vi "Geometry.vi"() -> ()   [LabVIEW 2018]
uses:
  <vilib>/Analysis/coordinate.llb/Euler Rotation Order.ctl
  <vilib>/imath/engines/lvmath2/RunTimeEngine/NodeEndStatement/NIMS_NodeEndStatement_Output.vi
  <instcachedir>/0/NIMS_NodeEndStatement_Output_53EC0D466D134D7ABD903AC30B43404B.lvgen/NIMS_NodeEndStatement_Output_53EC0D466D134D7ABD903AC30B43404B_005.vi
  <instcachedir>/0/NIMS_NodeEndStatement_Output_53EC0D466D134D7ABD903AC30B43404B.lvgen/NIMS_NodeEndStatement_Output_53EC0D466D134D7ABD903AC30B43404B_002.vi
  <vilib>/imath/engines/lvmath2/RunTimeEngine/ErrorHandling/NIMS_Finalize Error.vi
  <vilib>/imath/engines/lvmath2/RunTimeEngine/IndexRead/NIMS V(S).vi
  <instcachedir>/0/NIMS V(S)_0488751826AF41519A22953C041130DC.lvgen/NIMS V(S)_0488751826AF41519A22953C041130DC_000.vi
  <vilib>/imath/engines/lvmath2/RunTimeEngine/ErrorHandling/NIMS_Create Error From Enums.vi
  <vilib>/imath/engines/lvmath2/RunTimeEngine/ArithmeticOperatorToken/NIMS_ArithmeticOperator_multmx(M,CV)-internal.vi
  <instcachedir>/0/NIMS_ArithmeticOperator_multmx(M,CV)-internal_5287250D8D1D4A3E9F77F5DF08D432E0.lvgen/NIMS_ArithmeticOperator_multmx(M,CV)-internal_5287250D8D1D4A3E9F77F5DF08D432E0_001.vi
  <vilib>/imathl/engines/lvmath/Functions/Error Handling/Create Error.vi
  <vilib>/imath/engines/lvmath2/RunTimeEngine/ArithmeticOperatorToken/NIMS_ArithmeticOperator_multmx.vi
  <instcachedir>/0/NIMS_ArithmeticOperator_multmx_622CA76F9646436AB036D42A9A1CE0E6.lvgen/NIMS_ArithmeticOperator_multmx_622CA76F9646436AB036D42A9A1CE0E6_004.vi
  <vilib>/imath/engines/lvmath2/RunTimeEngine/ArithmeticOperatorToken/NIMS_ArithmeticOperator_multmx(M,CV).vi
  <instcachedir>/0/NIMS_ArithmeticOperator_multmx(M,CV)_2F1CD6A2FE4F4213A4AD1C901C2750F5.lvgen/NIMS_ArithmeticOperator_multmx(M,CV)_2F1CD6A2FE4F4213A4AD1C901C2750F5_000.vi
  <vilib>/imath/engines/lvmath2/RunTimeEngine/ArithmeticOperatorToken/NIMS_ArithmeticOperator_minus.vi
  <instcachedir>/0/NIMS_ArithmeticOperator_minus_C4D0373119CC411691B2E50DF2E09F22.lvgen/NIMS_ArithmeticOperator_minus_C4D0373119CC411691B2E50DF2E09F22_002.vi
  <vilib>/imath/engines/lvmath2/RunTimeEngine/IndexRead/NIMS M(S,S).vi
  <instcachedir>/0/NIMS M(S,S)_AC51E74150A542F7991B9634C66F3096.lvgen/NIMS M(S,S)_AC51E74150A542F7991B9634C66F3096_000.vi
  <instcachedir>/0/NIMS_NodeEndStatement_Output_53EC0D466D134D7ABD903AC30B43404B.lvgen/NIMS_NodeEndStatement_Output_53EC0D466D134D7ABD903AC30B43404B_001.vi
  <vilib>/imath/engines/lvmath2/RunTimeEngine/ArithmeticOperatorToken/NIMS_ArithmeticOperator_plus.vi
  <instcachedir>/0/NIMS_ArithmeticOperator_plus_DE670E32103C4C10ADF2A97367172B30.lvgen/NIMS_ArithmeticOperator_plus_DE670E32103C4C10ADF2A97367172B30_003.vi
  <instcachedir>/0/NIMS_NodeEndStatement_Output_53EC0D466D134D7ABD903AC30B43404B.lvgen/NIMS_NodeEndStatement_Output_53EC0D466D134D7ABD903AC30B43404B_004.vi
  <vilib>/imath/engines/lvmath2/RunTimeEngine/BuiltInFunctions/cross/NIMS_cross(GV,GV).vi
  <instcachedir>/0/NIMS_cross(GV,GV)_8E551EB9DC304C30866B49598818C259.lvgen/NIMS_cross(GV,GV)_8E551EB9DC304C30866B49598818C259_000.vi
  <vilib>/imath/engines/lvmath2/RunTimeEngine/BuiltInFunctions/inv/NIMS_inv(GM).vi
  <instcachedir>/0/NIMS_inv(GM)_A6DF8FE880224208AACFE4CF9F659502.lvgen/NIMS_inv(GM)_A6DF8FE880224208AACFE4CF9F659502_000.vi
  <vilib>/imath/engines/lvmath2/RunTimeEngine/ErrorHandling/NIMS_Error From Error Code.vi
  <vilib>/imath/engines/lvmath2/RunTimeEngine/BuiltInFunctions/cross/NIMS_cross(GM,GM,I32).vi
  <instcachedir>/0/NIMS_cross(GM,GM,I32)_0F6D45CF7D834A0BB6695B819A7F63BC.lvgen/NIMS_cross(GM,GM,I32)_0F6D45CF7D834A0BB6695B819A7F63BC_000.vi
  <vilib>/imath/engines/lvmath2/RunTimeEngine/IndexRead/NIMS M(S).vi
  <instcachedir>/0/NIMS M(S)_B826C018497E4940AE96BD27B540B6FB.lvgen/NIMS M(S)_B826C018497E4940AE96BD27B540B6FB_000.vi
  <vilib>/imath/engines/lvmath2/RunTimeEngine/BuiltInFunctions/norm/NIMS_norm(GM,DBL).vi
  <instcachedir>/0/NIMS_norm(GM,DBL)_14A9435485184B5E92336AF75A728284.lvgen/NIMS_norm(GM,DBL)_14A9435485184B5E92336AF75A728284_000.vi
  <vilib>/imath/engines/lvmath2/RunTimeEngine/IndexReplace/NIMS M(S,S)=S.vi
  <instcachedir>/0/NIMS M(S,S)=S_5DAF17B45D8A4C8588C7CF468644990A.lvgen/NIMS M(S,S)=S_5DAF17B45D8A4C8588C7CF468644990A_000.vi
  <vilib>/imath/engines/lvmath2/RunTimeEngine/NodeEndStatement/NIMS_NodeEndStatement_Get Vector.vi
  <instcachedir>/0/NIMS_NodeEndStatement_Get Vector_329D0992E87F49F089135171B7FC9327.lvgen/NIMS_NodeEndStatement_Get Vector_329D0992E87F49F089135171B7FC9327_001.vi
  <vilib>/imath/engines/lvmath/Functions/Error Handling/MergeErrorsWrapper.vi
  <vilib>/Analysis/NI_AALPro.lvlib
panel:
  out "rmg":dbl[](array[numeric])
  out "er 3":dbl(graph)
  out "er2":dbl(graph)
  out "er1":dbl(graph)
  out "Waveform Chart 3":dbl(graph)
  out "Waveform Chart 2":dbl(graph)
  out "Waveform Chart":dbl(graph)
  in  "Simulation Time(sec)":dbl
  in  "Physical Parameters":T1
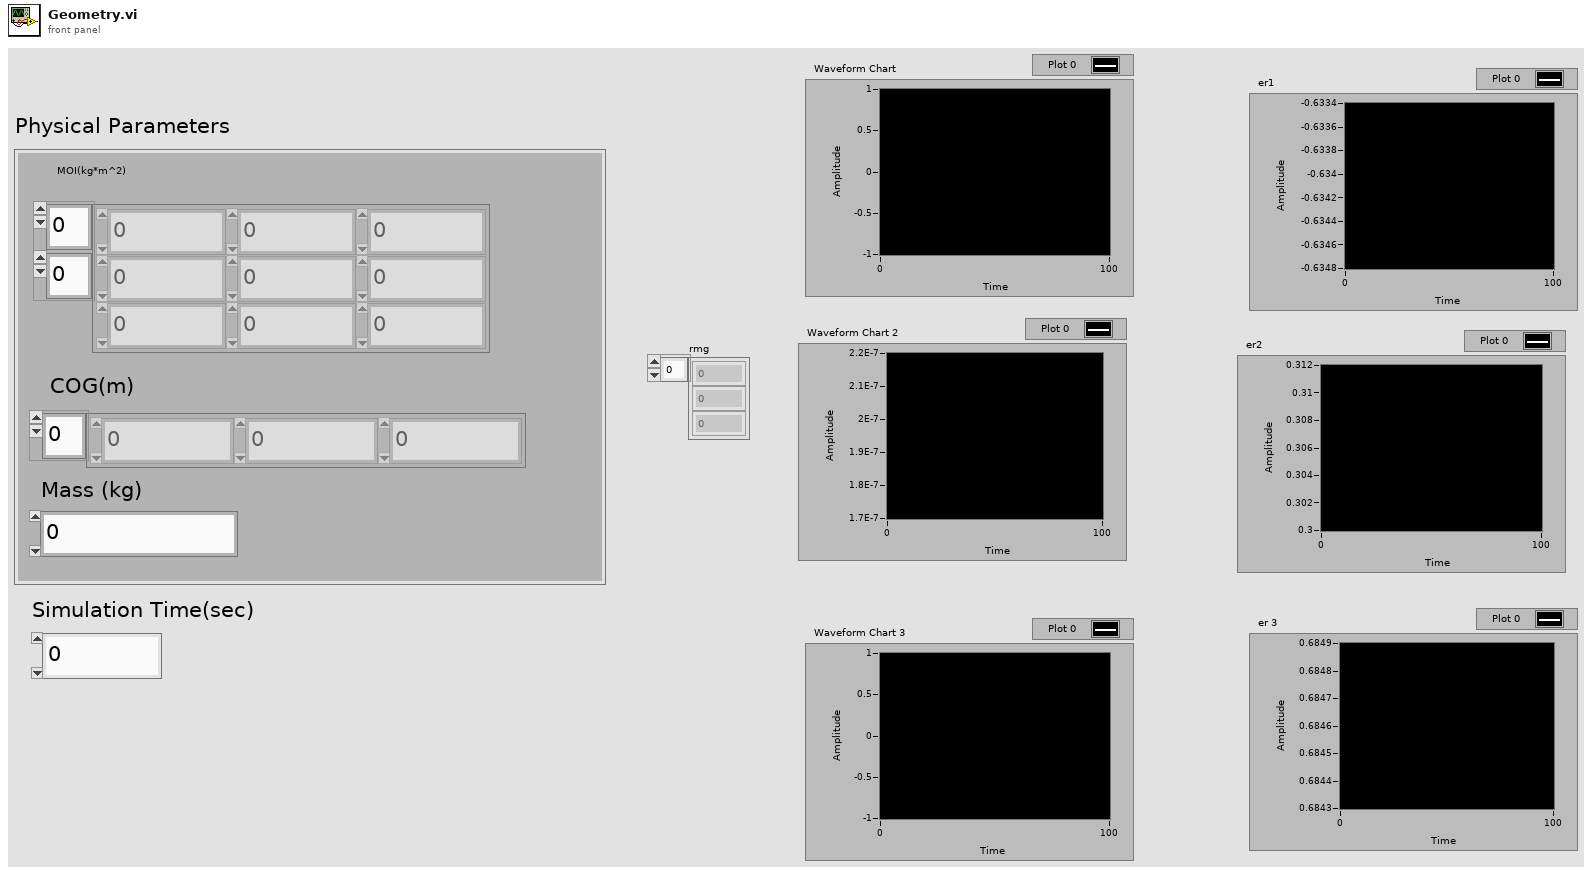
[diagram p1: front panel]
types:
  T1 = cluster{"Mass (kg)":dbl, "COG(m)":dbl[], "MOI(kg*m^2)":dbl[][]}
  T2 = typedef "NI_AALPro.lvlib/Euler Rotation Order.ctl" = u16
  T3 = cluster{"Direction Cosines":dbl[][], "Wd":dbl[], "W_dot_d":dbl[]}
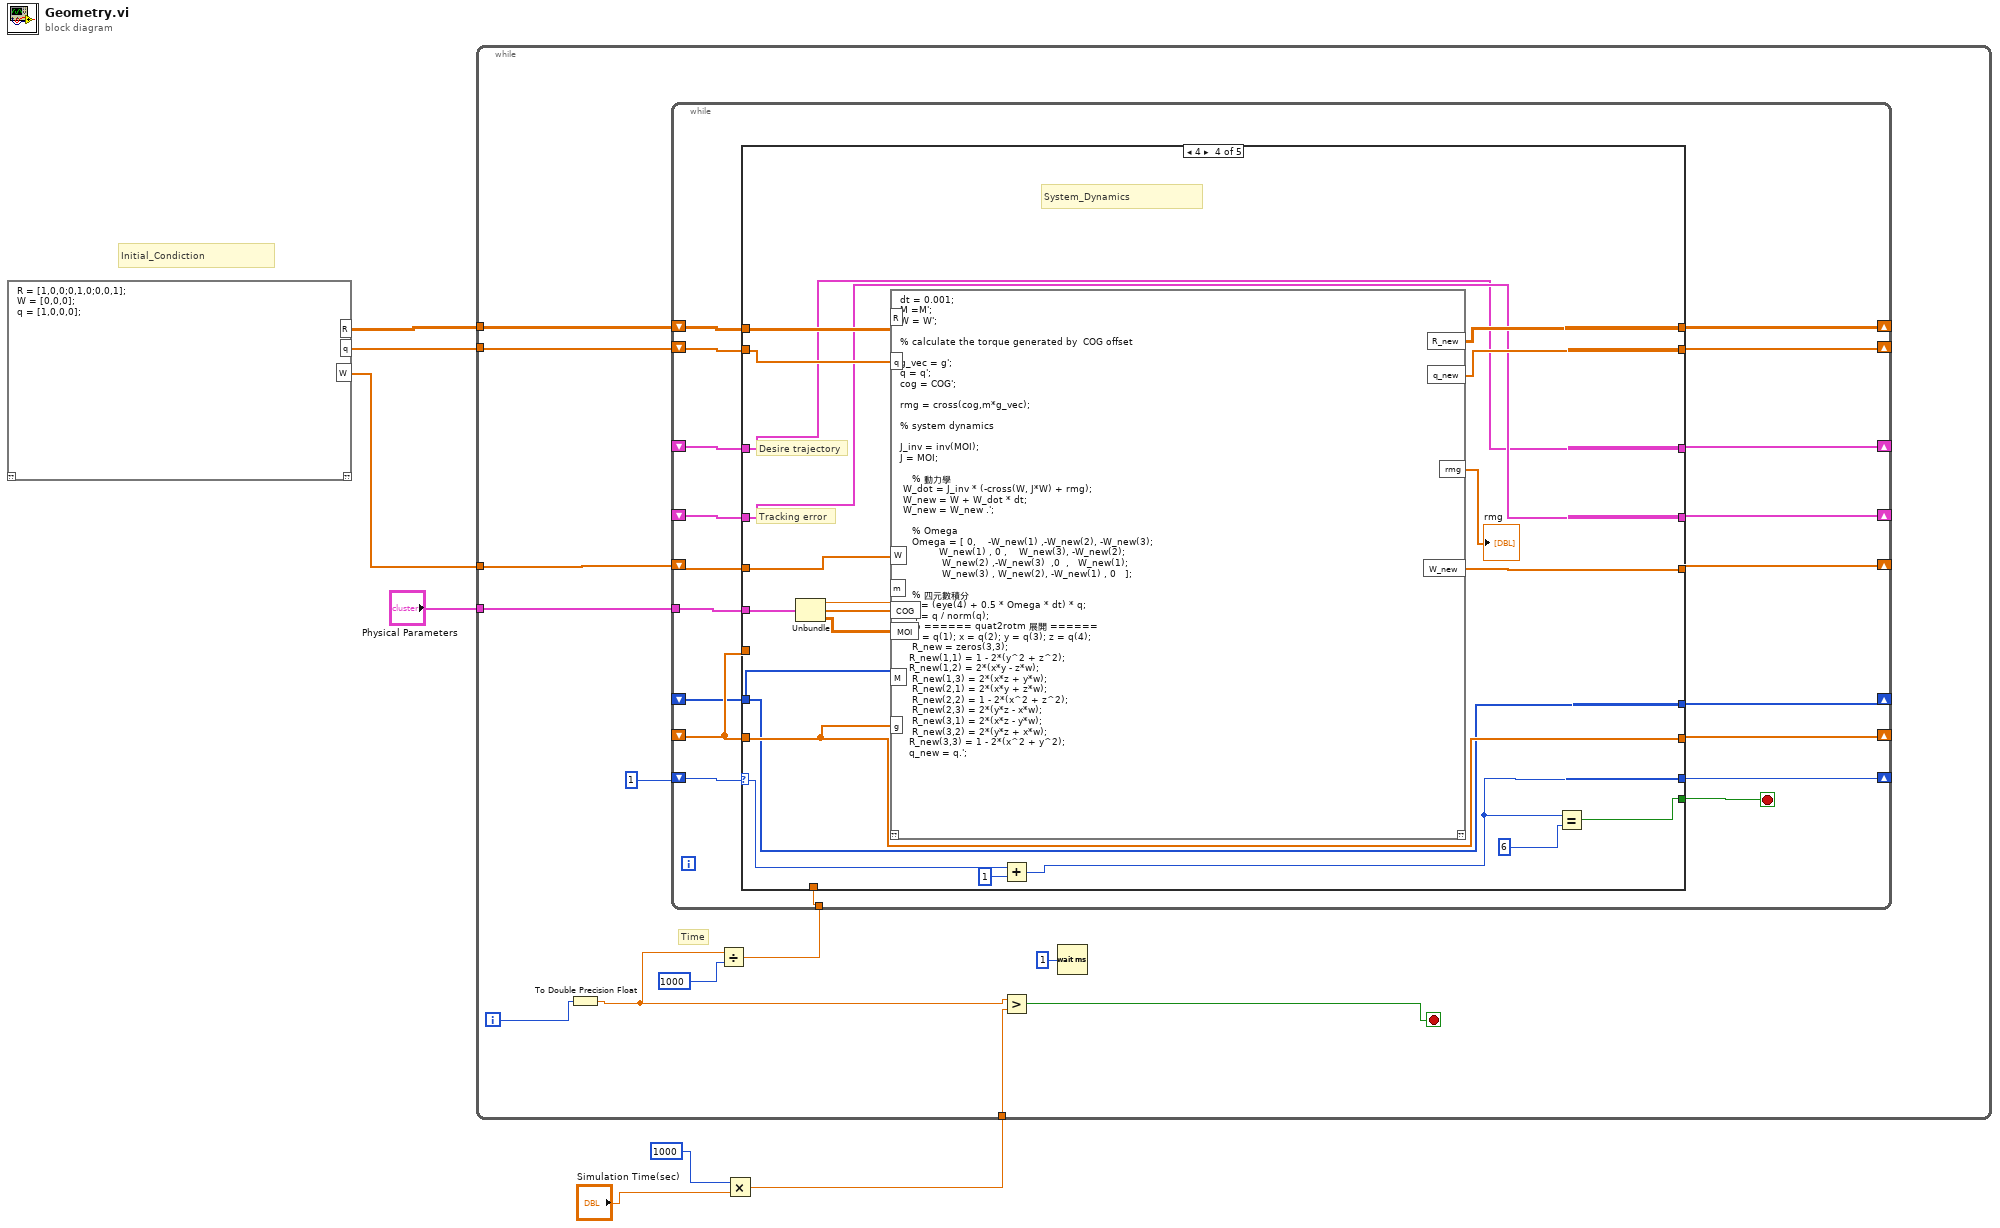
[diagram p0: block diagram]
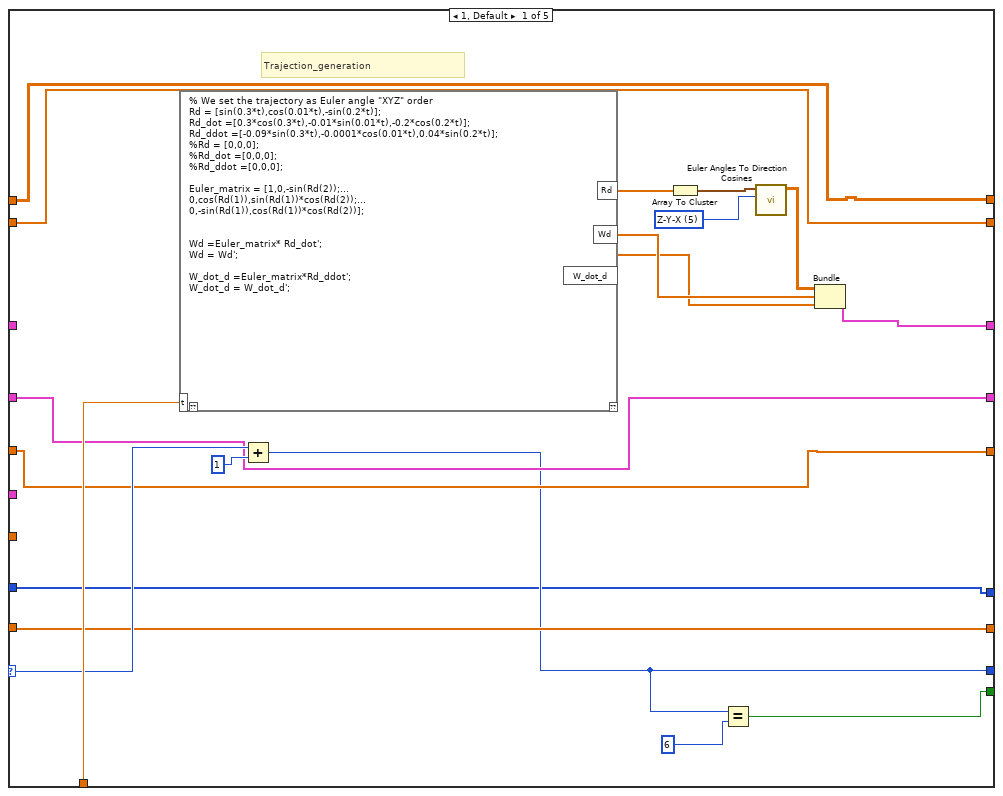
[diagram p2: hidden frame]
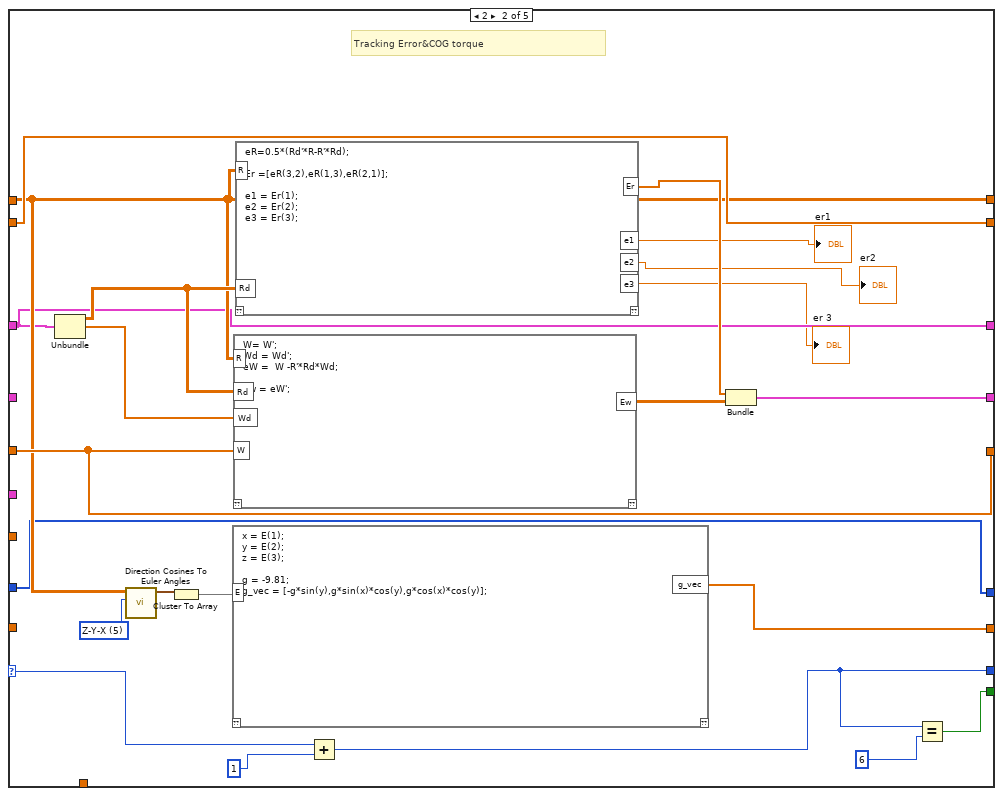
[diagram p3: hidden frame]
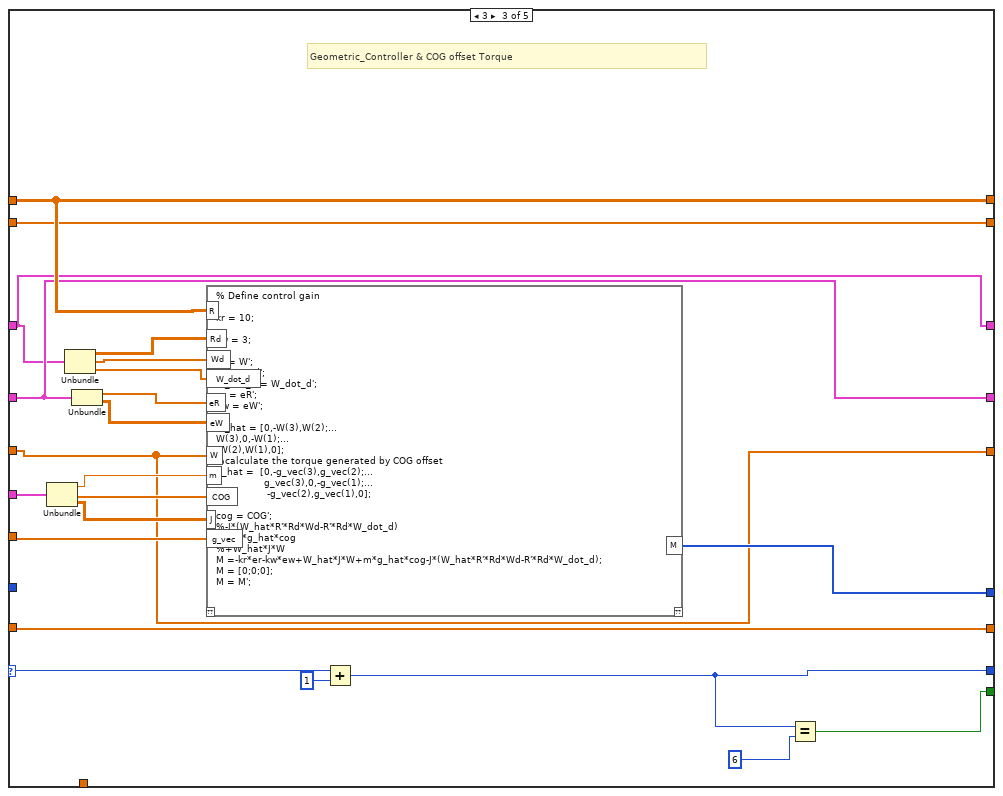
[diagram p4: hidden frame]
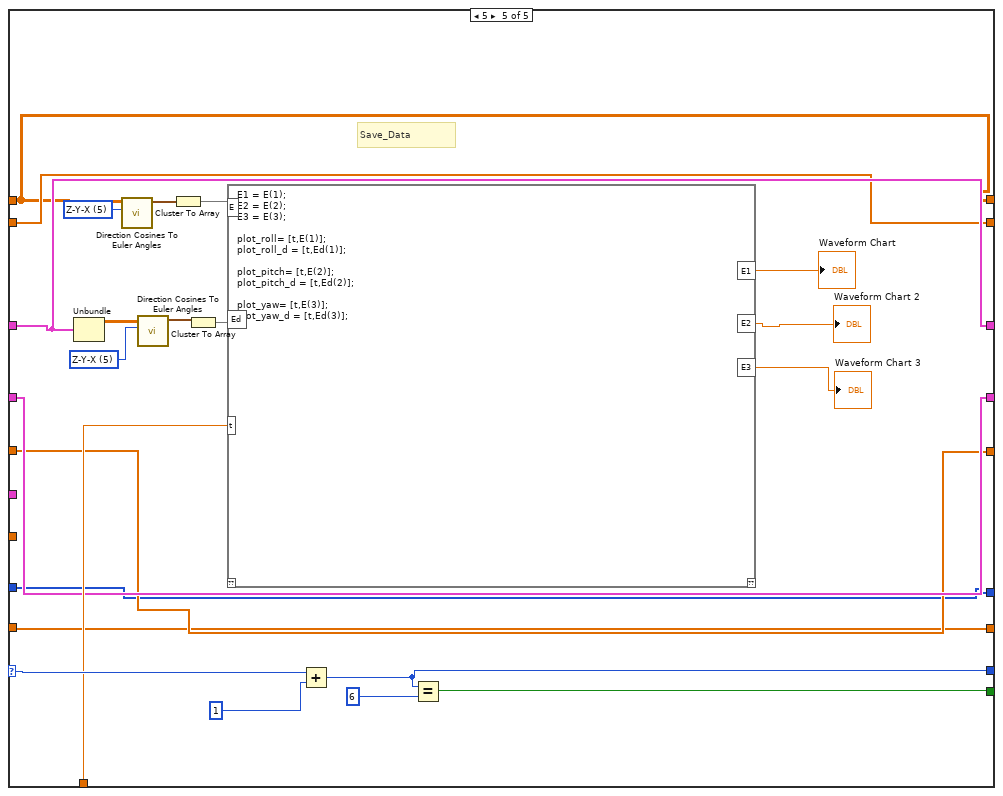
[diagram p5: hidden frame]
diagram:
  # "Initial_Condiction"
  n1 = mathscript code="R = [1,0,0;0,1,0;0,0,1];\nW = [0,0,0];\nq = [1,0,0,0];"() -> ("R"=w4:dbl[][], "W"=w3:dbl[], "q"=w1:dbl[])  [unwired: 1 in, 1 out]
  n2 = Multiply(x=1000, y="Simulation Time(sec)") -> (x*y=w5:dbl)
  n3 = while {
    tunnel: w5 -> [w17]
    tunnel: w4 -> [w12]
    tunnel: w3 -> [w11]
    tunnel: "Physical Parameters" -> [w10]
    tunnel: w1 -> [w9]
    i -> [w15]
    stop <- w18 stop-if-true
    # "Time"
    n4 = To Double Precision Float(number=w15) -> (double precision float=w13:dbl)
    n5 = Divide(x=w13, y=1000) -> (x/y=w14:dbl)
    n6 = while {
      shift-right: [w36] -> _
      shift-left: 1 -> [w38]
      tunnel: w14 -> [w37]
      shift-right: [w35] -> _
      shift-left: _ -> [w34]
      shift-right: [w33] -> _
      shift-left: _ -> [w32]
      shift-right: [w29] -> _
      shift-left: w12 -> [w31]
      shift-right: [w28] -> _
      shift-left: w11 -> [w30]
      shift-right: [w27] -> _
      shift-left: _ -> [w26]
      tunnel: w10 -> [w25]
      shift-right: [w24] -> _
      shift-left: _ -> [w23]
      shift-right: [w21] -> _
      shift-left: w9 -> [w22]
      stop <- w20 stop-if-true
      n7 = case shown="4" w38 {
        selector: w38 -> [w53 w262 w580 w896 w1606]
        tunnel: w37 -> [w57 _ _ _ w1595]
        tunnel: [w54 w255 w576 w889 w1594] -> w35
        tunnel: [w42 w253 w574 w886 w1587] -> w36
        tunnel: w34 -> [_ w255 w576 w889 w1594]
        tunnel: [w45 w264 w577 w890 w1593] -> w33
        tunnel: w32 -> [w45 _ w577 w890 w1593]
        tunnel: w31 -> [w39 w256 w582 w901 w1588]
        tunnel: w30 -> [w46 w263 w581 w902 w1592]
        tunnel: [w39 w256 w582 w893 w1588] -> w29
        tunnel: [w46 w263 w581 w891 w1592] -> w28
        tunnel: [w44 w258 w591 w888 w1591] -> w27
        tunnel: w26 -> [_ _ w592 _ _]
        tunnel: w26 -> [w44 _ w591 w888 w1591]
        tunnel: w25 -> [_ _ w590 w900 _]
        tunnel: [w40 w251 w583 w887 w1590] -> w24
        tunnel: w23 -> [w40 w251 _ w887 w1590]
        tunnel: w22 -> [w47 w257 w578 w894 w1589]
        tunnel: [w47 w257 w578 w892 w1589] -> w21
        tunnel: [w41 w252 w573 w884 w1603] -> w20
        frame 1, Default {
          w48 = T2 5 items=["X-Y-Z", "X-Z-Y", "Y-X-Z", "Y-Z-X", "Z-X-Y", "Z-Y-X", "X-Y-X", "X-Z-X", "Y-X-Y", "Y-Z-Y", "Z-X-Z", "Z-Y-Z"] ("rotation order")
          # "Trajection_generation"
          n8 = mathscript code="% We set the trajectory as Euler angle \"XYZ\" order\nRd = [sin(0.3*t),cos(0.01*t),-sin(0.2*t)];\nRd_dot =[0.3*cos(0.3*t),-0.01*sin(0.01*t),-0.2*cos(0.2*t)];\nRd_ddot =[-0.09*sin(0.3*t),-0.0001*cos(0.01*t),0.04*sin(0.2*t)];\n%Rd = [0,0,0];\n%Rd_dot =[0,0,0];\n%Rd_ddot =[0,0,0];\n\nEuler_matrix = [1,0,-sin(Rd(2));...\n0,cos(Rd(1)),sin(Rd(1))*cos(Rd(2));...\n0,-sin(Rd(1)),cos(Rd(1))*cos(Rd(2))];\n\n\nWd =Euler_matrix* Rd_dot';\nWd = Wd';\n\nW_dot_d =Euler_matrix*Rd_ddot';\nW_dot_d = W_dot_d';"("t"=w57) -> ("Rd"=w51:dbl[], "Wd"=w56:dbl[], "W_dot_d"=w55:dbl[])  [unwired: 1 in, 1 out]
          n9 = Add(x=w53, y=1) -> (x+y=w42:i32)
          n10 = Array To Cluster(array=w51) -> (cluster=w50:cluster{"Rd[0]":dbl, "Rd[1]":dbl, "Rd[2]":dbl})
          n11 = Equal?(x=w42, y=6) -> (x = y?=w41:bool)
          n12 = call <vilib>:"Euler Angles To Direction Cosines.vi"("rotation order"=w48, "Euler Angles"=w50) -> ("Direction Cosines"=w49:dbl[][])  [unwired: 8 in, 1 out]
          n13 = Bundle("Direction Cosines"=w49, "Wd"=w56, "W_dot_d"=w55) -> (w54:T3)  [unwired: 1 in]
        }
        frame 2 {
          w260 = T2 5 items=["X-Y-Z", "X-Z-Y", "Y-X-Z", "Y-Z-X", "Z-X-Y", "Z-Y-X", "X-Y-X", "X-Z-X", "Y-X-Y", "Y-Z-Y", "Z-X-Z", "Z-Y-Z"] ("rotation order")
          # "Tracking Error&COG torque"
          n14 = Unbundle(w255) -> ("Direction Cosines"=w268:dbl[][], "Wd"=w267:dbl[])  [unwired: 1 out]
          n15 = call <vilib>:"Direction Cosines To Euler Angles.vi"("rotation order"=w260, "Direction Cosines"=w256) -> ("Euler Angles"=w247:cluster{"phi":dbl, "theta":dbl, "psi":dbl})  [unwired: 8 in, 1 out]
          n16 = Cluster To Array(cluster=w247) -> (array=w259:dbl[])
          n17 = mathscript code="x = E(1);\ny = E(2);\nz = E(3);\n\ng = -9.81;\ng_vec = [-g*sin(y),g*sin(x)*cos(y),g*cos(x)*cos(y)];"("E"=w259) -> ("g_vec"=w258:dbl[])  [unwired: 1 in, 1 out]
          n18 = mathscript code="W= W';\nWd = Wd';\neW =  W -R'*Rd*Wd;\n\nEw = eW';"("Rd"=w268, "Wd"=w267, "W"=w263, "R"=w256) -> ("Ew"=w265:dbl[][])  [unwired: 1 in, 1 out]
          n19 = mathscript code="eR=0.5*(Rd'*R-R'*Rd);\n\nEr =[eR(3,2),eR(1,3),eR(2,1)];\n\ne1 = Er(1);\ne2 = Er(2);\ne3 = Er(3);"("Rd"=w268, "R"=w256) -> ("Er"=w266:dbl[], "e1"=→"er1":dbl, "e2"=→"er2":dbl, "e3"=→"er 3":dbl)  [unwired: 1 in, 1 out]
          n20 = Add(x=w262, y=1) -> (x+y=w253:i32)
          n21 = Bundle("Er"=w266, "Ew"=w265) -> (w264:cluster{"Er":dbl[], "Ew":dbl[][]})  [unwired: 1 in]
          n22 = Equal?(x=w253, y=6) -> (x = y?=w252:bool)
        }
        frame 3 {
          # "Geometric_Controller & COG offset Torque"
          n23 = Unbundle(w590) -> ("Mass (kg)"=w589:dbl, "COG(m)"=w587:dbl[], "MOI(kg*m^2)"=w588:dbl[][])
          n24 = Unbundle(w576) -> ("Direction Cosines"=w586:dbl[][], "Wd"=w585:dbl[], "W_dot_d"=w584:dbl[])
          n25 = Unbundle(w577) -> ("Er"=w594:dbl[], "Ew"=w593:dbl[][])
          n26 = mathscript code="% Define control gain\n\nkr = 10;\n\nkw = 3;\n\nW = W';\nWd = Wd';\nW_dot_d = W_dot_d';\ner = eR';\new = eW';\n\nW_hat = [0,-W(3),W(2);...\nW(3),0,-W(1);...\n-W(2),W(1),0];\n%calculate the torque generated by COG offset \ng_hat =  [0,-g_vec(3),g_vec(2);...\n                g_vec(3),0,-g_vec(1);...\n                 -g_vec(2),g_vec(1),0];\n\ncog = COG';\n%-J*(W_hat*R'*Rd*Wd-R'*Rd*W_dot_d)\n%+m*g_hat*cog\n%+W_hat*J*W\nM =-kr*er-kw*ew+W_hat*J*W+m*g_hat*cog-J*(W_hat*R'*Rd*Wd-R'*Rd*W_dot_d);\nM = [0;0;0];\nM = M';"("W"=w581, "eR"=w594, "eW"=w593, "R"=w582, "J"=w588, "g_vec"=w592, "m"=w589, "COG"=w587, "Rd"=w586, "Wd"=w585, "W_dot_d"=w584) -> ("M"=w583:i32[])  [unwired: 1 in, 1 out]
          n27 = Add(x=w580, y=1) -> (x+y=w574:i32)
          n28 = Equal?(x=w574, y=6) -> (x = y?=w573:bool)
        }
        frame 4 {
          # "Tracking error"
          # "Desire trajectory"
          # "System_Dynamics"
          n29 = Unbundle(w900) -> ("Mass (kg)"=w899:dbl, "COG(m)"=w898:dbl[], "MOI(kg*m^2)"=w897:dbl[][])
          n30 = mathscript code="dt = 0.001;\nM =M';\nW = W';\n\n% calculate the torque generated by  COG offset\n\ng_vec = g';\nq = q';\ncog = COG';\n\nrmg = cross(cog,m*g_vec);\n\n% system dynamics\n\nJ_inv = inv(MOI);\nJ = MOI;\n\n    % 動力學\n W_dot = J_inv * (-cross(W, J*W) + rmg);\n W_new = W + W_dot * dt;\n W_new = W_new .';\n\n    % Omega\n    Omega = [ 0,    -W_new(1) ,-W_new(2), -W_new(3);\n             W_new(1) , 0 ,    W_new(3), -W_new(2);\n              W_new(2) ,-W_new(3)  ,0  ,   W_new(1);\n              W_new(3) , W_new(2), -W_new(1) , 0   ];\n\n    % 四元數積分\n    q = (eye(4) + 0.5 * Omega * dt) * q;\n    q = q / norm(q);\n    % ====== quat2rotm 展開 ======\n    w = q(1); x = q(2); y = q(3); z = q(4);\n    R_new = zeros(3,3);\n   R_new(1,1) = 1 - 2*(y^2 + z^2);\n   R_new(1,2) = 2*(x*y - z*w);\n    R_new(1,3) = 2*(x*z + y*w);\n    R_new(2,1) = 2*(x*y + z*w);\n    R_new(2,2) = 1 - 2*(x^2 + z^2);\n    R_new(2,3) = 2*(y*z - x*w);\n    R_new(3,1) = 2*(x*z - y*w);\n    R_new(3,2) = 2*(y*z + x*w);\n   R_new(3,3) = 1 - 2*(x^2 + y^2);\n   q_new = q.';"("W"=w902, "R"=w901, "m"=w899, "COG"=w898, "MOI"=w897, "g"=w888, "M"=w887, "q"=w894) -> ("R_new"=w893:dbl[][], "q_new"=w892:dbl[], "W_new"=w891:dbl[], "rmg"=→"rmg":dbl[])  [unwired: 1 in, 1 out]
          n31 = Add(x=w896, y=1) -> (x+y=w886:i32)
          n32 = Equal?(x=w886, y=6) -> (x = y?=w884:bool)
        }
        frame 5 {
          w1598 = T2 5 items=["X-Y-Z", "X-Z-Y", "Y-X-Z", "Y-Z-X", "Z-X-Y", "Z-Y-X", "X-Y-X", "X-Z-X", "Y-X-Y", "Y-Z-Y", "Z-X-Z", "Z-Y-Z"] ("rotation order")
          w1602 = T2 5 items=["X-Y-Z", "X-Z-Y", "Y-X-Z", "Y-Z-X", "Z-X-Y", "Z-Y-X", "X-Y-X", "X-Z-X", "Y-X-Y", "Y-Z-Y", "Z-X-Z", "Z-Y-Z"] ("rotation order")
          # "Save_Data"
          n33 = Unbundle(w1594) -> ("Direction Cosines"=w1599:dbl[][])  [unwired: 2 out]
          n34 = call <vilib>:"Direction Cosines To Euler Angles.vi"("rotation order"=w1602, "Direction Cosines"=w1588) -> ("Euler Angles"=w1601:cluster{"phi":dbl, "theta":dbl, "psi":dbl})  [unwired: 8 in, 1 out]
          n35 = call <vilib>:"Direction Cosines To Euler Angles.vi"("rotation order"=w1598, "Direction Cosines"=w1599) -> ("Euler Angles"=w1597:cluster{"phi":dbl, "theta":dbl, "psi":dbl})  [unwired: 8 in, 1 out]
          n36 = Cluster To Array(cluster=w1601) -> (array=w1600:dbl[])
          n37 = Cluster To Array(cluster=w1597) -> (array=w1596:dbl[])
          n38 = mathscript code="E1 = E(1);\nE2 = E(2);\nE3 = E(3);\n\nplot_roll= [t,E(1)];\nplot_roll_d = [t,Ed(1)];\n\nplot_pitch= [t,E(2)];\nplot_pitch_d = [t,Ed(2)];\n\nplot_yaw= [t,E(3)];\nplot_yaw_d = [t,Ed(3)];"("E"=w1600, "Ed"=w1596, "t"=w1595) -> ("E1"=→"Waveform Chart":dbl, "E2"=→"Waveform Chart 2":dbl, "E3"=→"Waveform Chart 3":dbl)  [unwired: 1 in, 1 out]
          n39 = Add(x=w1606, y=1) -> (x+y=w1587:i32)
          n40 = Equal?(x=w1587, y=6) -> (x = y?=w1603:bool)
        }
      }
    }
    n41 = Greater?(x=w13, y=w17) -> (0:w18:bool)
    n42 = Wait (ms)(milliseconds to wait=u32 1) -> ()  [unwired: 1 out]
  }
